vi "Temperature Limit.vi"() -> ()   [LabVIEW 2012]
doc: "该VI可仿真温度采集，绘制温度图形，并通知用户温度是否超出范围。"
panel:
  in  "开始":bool
  in  "△t(ms)":i32(slide)=400 scale=50.0..500.0
  in  "停止":bool
  in  "上限":dbl=28.0 format="%.2f"
  out "温度":cluster{"Temperature":dbl, "High Limit":dbl}(graph)={"Temperature"=85.88749999999999, "High Limit"=80.0}
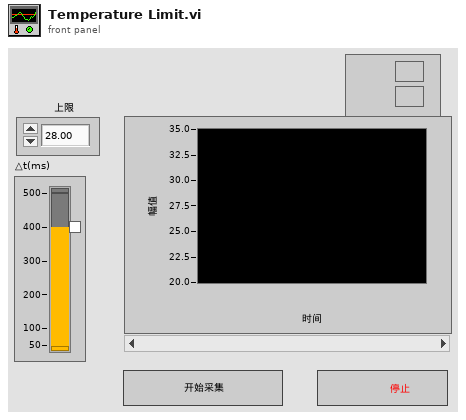
[diagram p1: front panel]
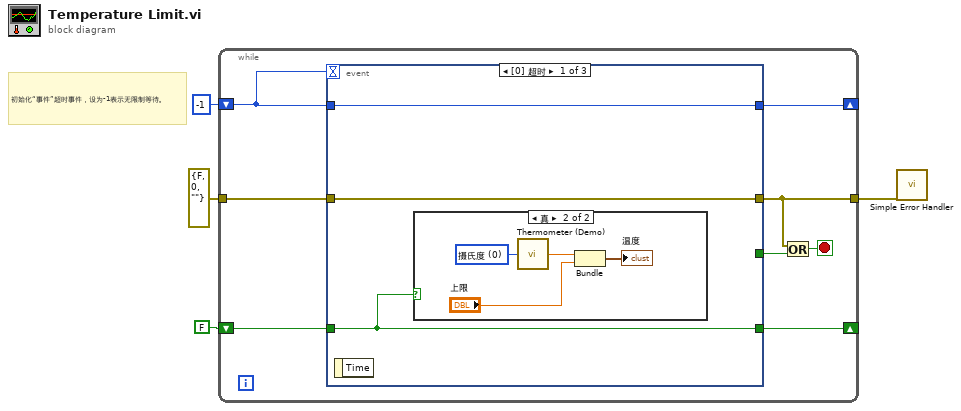
[diagram p0: block diagram]
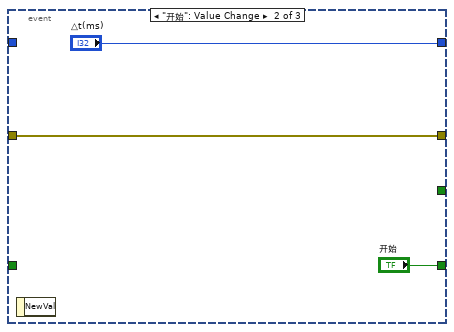
[diagram p3: hidden frame]
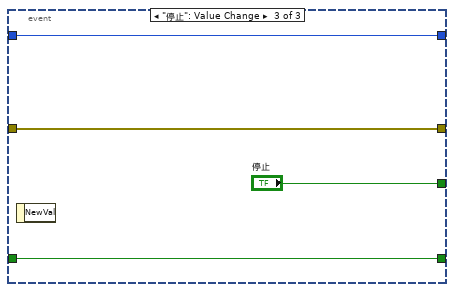
[diagram p4: hidden frame]
diagram:
  # "初始化“事件”超时事件，设为-1表示无限制等待。"
  n1 = while {
    tunnel: cluster{"状态":bool, "代码":i32, "源":string} {"状态"=FALSE, "代码"=0, "源"=""} ("错误输出") -> [w12]
    tunnel: [w10] -> w3
    shift-right: [w8] -> _
    shift-left: FALSE ("开始") -> [w7]
    shift-right: [w6] -> _
    shift-left: -1 ("△t(ms)") -> [w5]
    stop <- w11 stop-if-true
    n2 = event shown="[0] 超时" {
      selector: _ -> [_ _ _]
      dyn-events: _ -> [_ _ _]
      timeout: w5 -> [_ _ _]
      tunnel: [_ _ "停止"] -> w9
      tunnel: w12 -> [w15 w20 w25]
      tunnel: [w15 w20 w25] -> w10
      tunnel: [w13 "开始" w24] -> w8
      tunnel: w7 -> [w13 _ w24]
      tunnel: [w14 "△t(ms)" w23] -> w6
      tunnel: w5 -> [w14 _ w23]
      event Timeout {
        n3 = event-data ("事件数据节点")() -> ()  [unwired: 1 in, 1 out]
        n4 = case shown="真" w13 {
          frame False {
          }
          frame True {
            w16 = u16 0 items=["摄氏度", "华氏度"] ("单位（0：摄氏度）")
            n5 = call "Thermometer (Demo).vi"("单位（0：摄氏度）"=w16) -> ("温度值"=w17:dbl)
            n6 = Bundle ("捆绑")("温度值"=w17, "上限"="上限") -> (→"温度":cluster{"温度值":dbl, "上限":dbl})  [unwired: 1 in]
          }
        }
      }
      event "开始": Value Change {
        n7 = event-data ("事件数据节点")() -> ()  [unwired: 1 in, 1 out]
      }
      event "停止": Value Change {
        n8 = event-data ("事件数据节点")() -> ()  [unwired: 1 in, 1 out]
      }
    }
    n9 = Or ("或")(x=w10, y=w9) -> (x .or. y?=w11:bool)
  }
  n10 = call <vilib>:"Simple Error Handler.vi"("error in (no error)"=w3) -> ()  [unwired: 4 in, 5 out]
